vi "InsertObjType.vi"(0 "reference in":refnum<class "Logger.lvclass">, 11 "error in (no error)":errorcluster) -> (4 "reference out":refnum<class "Logger.lvclass">, 14 "dt (ms)":u32, 15 "error out":errorcluster)   [LabVIEW 2019, in "Logger.lvclass"]
uses:
  Logger.lvclass
  ObjType.ctl
  Logger.lvclass/Logger.ctl
  392f7031-4897-4389-b682-77fa04bcb28f.vi
  9e415a43-db33-4f06-8781-9fdd0a489df8.vi
  DatabaseInterface_class/DatabaseInterface.lvclass
panel:
  in  "ObjType":T1
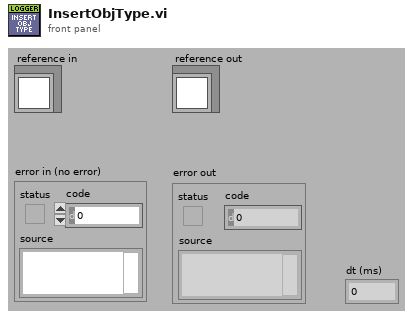
[diagram p1: front panel]
types:
  T1 = typedef "Logger.lvclass/ObjType.ctl" = enum16{"Procces", "Device", "Signal", "DI", "DO", "DA", "AI", "AO", "AA"}
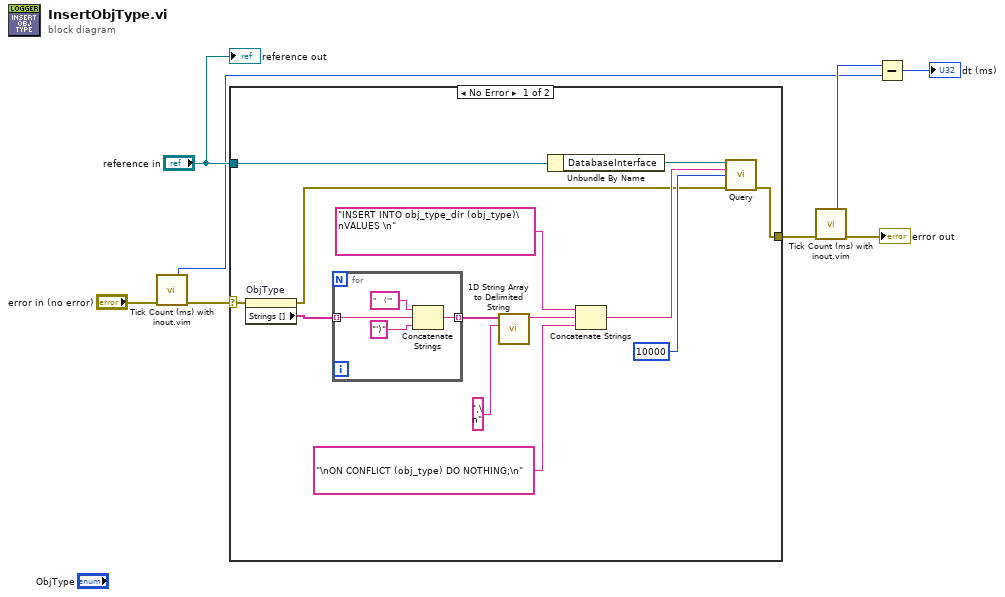
[diagram p0: block diagram]
diagram:
  n1 = call "Tick Count (ms) with inout.vim"("in"="error in (no error)") -> ("millisecond timer value"=w1:u32, "out"=w4:errorcluster)  [unwired: 12 in, 1 out]
  n2 = case shown="No Error" w4 {
    selector: w4 -> [w17 w26]
    tunnel: [w16 w26] -> w7
    tunnel: "reference in" -> [w10 _]
    frame No Error {
      n3 = property on="ObjType" class="Enum (strict)"(error in=w17) -> (error out=w9:errorcluster, "Strings []"=w19:string[])  [unwired: 1 in, 1 out]
      n4 = for {
        tunnel: w19 -> [w24] mode=indexing
        tunnel: [w22] -> w15 mode=indexing
        n5 = Concatenate Strings("    ('" ("format string"), w24, "')" ("format string")) -> (w22:string)
      }
      n6 = call <vilib>:"1D String Array to Delimited String.vi"("delimiter"=",\n", "string array"=w15) -> ("delimited string"=w13:string)  [unwired: 9 in]
      n7 = Unbundle By Name(w10) -> ("DatabaseInterface"=w20:refnum<class "DatabaseInterface.lvclass">)
      n8 = Concatenate Strings("INSERT INTO obj_type_dir (obj_type)\nVALUES \n" ("format string"), w13, "\nON CONFLICT (obj_type) DO NOTHING;\n" ("format string")) -> (w11:string)
      n9 = call-dynamic "Query.vi"("reference in"=w20, "Query"=w11, "Timeout"=10000, "error in (no error)"=w9) -> ("error out"=w16:errorcluster)  [unwired: 9 in, 2 out]
    }
    frame Error {
    }
  }
  n10 = call "Tick Count (ms) with inout.vim"("in"=w7) -> ("millisecond timer value"=w2:u32, "out"=→"error out":errorcluster)  [unwired: 12 in, 1 out]
  n11 = Subtract(x=w2, y=w1) -> (x-y=→"dt (ms)":u32)
  "reference out" <- "reference in"
